vi "Message.vi"() -> (0 "error out":errorcluster)   [LabVIEW 2017, in "Transparent Assertions.Tests.lvlib" / "Assert True.lvlib"]
uses:
  Assert True.lvlib
  src/Transparent Assertions/Transparent Assertions.lvlib
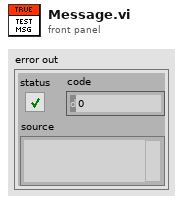
[diagram p1: front panel]
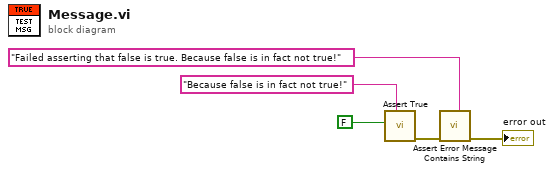
[diagram p0: block diagram]
diagram:
  n1 = call "Assert True.vi"("Message (\"\")"="Because false is in fact not true!" ("Message (\"\")"), "Condition"=FALSE) -> ("error out"=w4:errorcluster)  [unwired: 9 in]
  n2 = call "Assert Error Message Contains String.vi"("Expected"="Failed asserting that false is true. Because false is in fact not true!" ("y"), "error in (no error)"=w4) -> ("error out"=→"error out":errorcluster)  [unwired: 9 in]
